vi "Init.vi"(8 "error in (no error)":errorcluster, 10 "Address":string, 11 "ZWO_ASI in":refnum<class "ZWO_ASI.lvclass">) -> (0 "error out":errorcluster, 3 "ZWO_ASI out":refnum<class "ZWO_ASI.lvclass">)   [LabVIEW 2023, in "ZWO_ASI.lvlib" / "ZWO_ASI.lvclass"]
uses:
  ZWO_ASI.lvclass
  ZWO_ASI.lvclass/ZWO_ASI.ctl
  <userlib>/ASICamera2_no_err/ASICamera2_no_err.lvlib
  InitDeinitComm Messages/InitDone Msg/InitDone Msg.lvclass
  <vilib>/ActorFramework/Actor/Actor.lvclass
  Applications/National Instruments/LabVIEW 2023 64-bit/vi.lib/ActorFramework/Actor/Actor.lvclass
  Users/alexandrosspiliotis/Documents/ZWO_ASI/ZWO_ASI/ZWO_ASI.lvclass
  Users/alexandrosspiliotis/Documents/TranslationStage/InitDeinit/InitDeinit.lvclass
  Users/alexandrosspiliotis/Documents/OrcaLV/ImagingDevice/ImagingDevice.lvclass
panel:
  in  "Address":T1
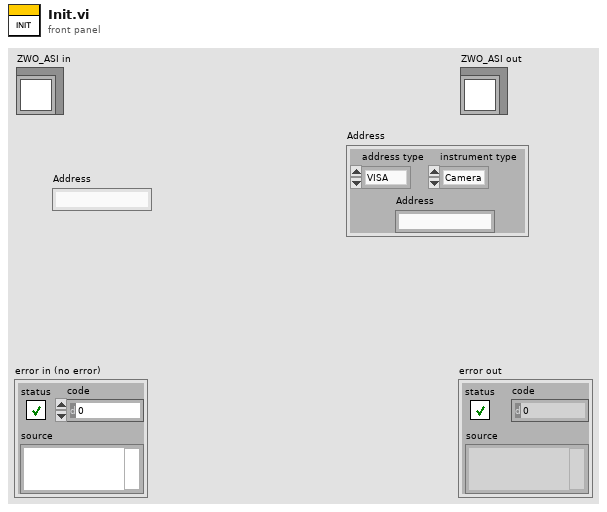
[diagram p1: front panel]
types:
  T1 = cluster{"address type":enum16{"VISA", "Index"}, "Address":string, "instrument type":enum16{"Camera", "Stepper"}}
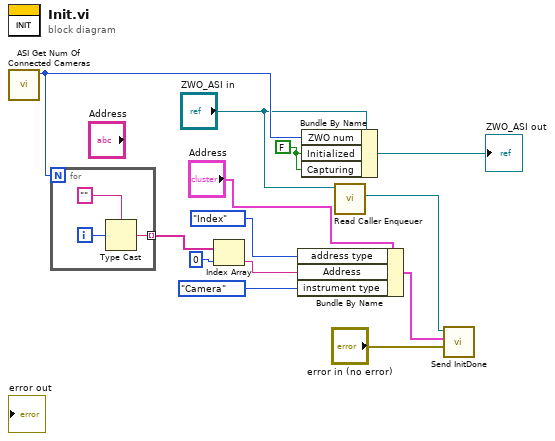
[diagram p0: block diagram]
diagram:
  w12 = FALSE ("Initialized")
  n1 = call <userlib>:"ASI Get Num Of Connected Cameras.vi"() -> ("function return"=w11:i32)  [unwired: 11 in]
  n2 = for {
    N: w11 -> [_]
    tunnel: [w14] -> w4 mode=indexing
    i -> [w15]
    n3 = Type Cast(type="", x=w15) -> (*(type *) &x=w14:string)
  }
  n4 = Index Array(array=w4, index=0) -> (element=w2:string)
  n5 = Bundle By Name(cluster="Address", "address type"=enum16{"VISA", "Index"}."Index", "Address"=w2, "instrument type"=enum16{"Camera", "Stepper"}."Camera" ("Camera.instrument type")) -> (w1:T1)
  n6 = Bundle By Name(cluster="ZWO_ASI in", "ZWO num"=w11, "Initialized"=w12, "Capturing"=w12) -> (→"ZWO_ASI out":refnum<class "ZWO_ASI.lvclass">)
  n7 = call <vilib>:"Read Caller Enqueuer.vi"("Actor"="ZWO_ASI in") -> ("Caller Enqueuer"=w9:refnum<class "Message Enqueuer.lvclass">)  [unwired: 10 in]
  n8 = call "Send InitDone.vi"("instr error"="error in (no error)", "Address"=w1, "Message Enqueuer"=w9) -> ()  [unwired: 7 in, 2 out]
